vi "Destroy RawDataQs.vi"(8 "error in (no error)":errorcluster, 11 "DAQ":refnum<class "DAQ.lvclass">) -> (0 "error out":errorcluster, 3 "DAQ":refnum<class "DAQ.lvclass">)   [LabVIEW 2022 SP3, in "DAQ.lvclass"]
doc: "Developed by Kevin Thompson\nkevin@thompsonengineering.net\n\nCopyright 2018-2020\nThompson Engineering, LLC"
uses:
  DAQ.lvclass
  DAQ.lvclass/DAQ.ctl
  Process/ProcessSupport/TD local raw AI Data--cluster.ctl
  Support/DataQueues/DataTypes/DataQ SelectType--enum.ctl
  Support/DataQueues/DataQueues.lvclass
  DataTypes/Dependency--cluster.ctl
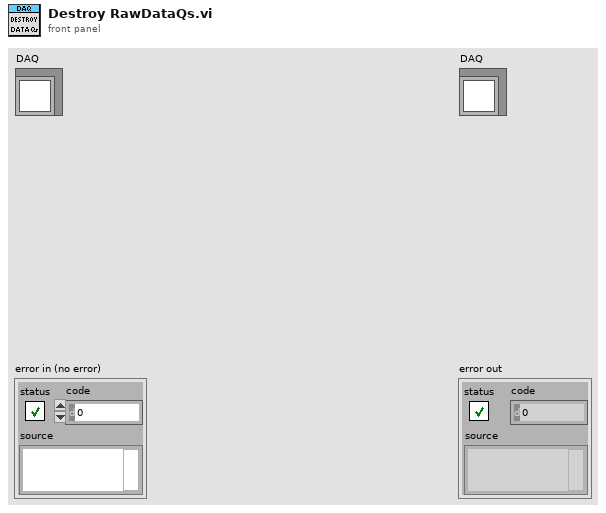
[diagram p1: front panel]
types:
  T1 = typedef "DAQ.lvclass/Dependency--cluster.ctl" = cluster{"DataQueues":refnum<class "DataQueues.lvclass">}
  T2 = typedef "DataQueues.lvclass/DataQ SelectType--enum.ctl" = enum16{"MainProcess", "LogEngine", "LocalDAQThread"}
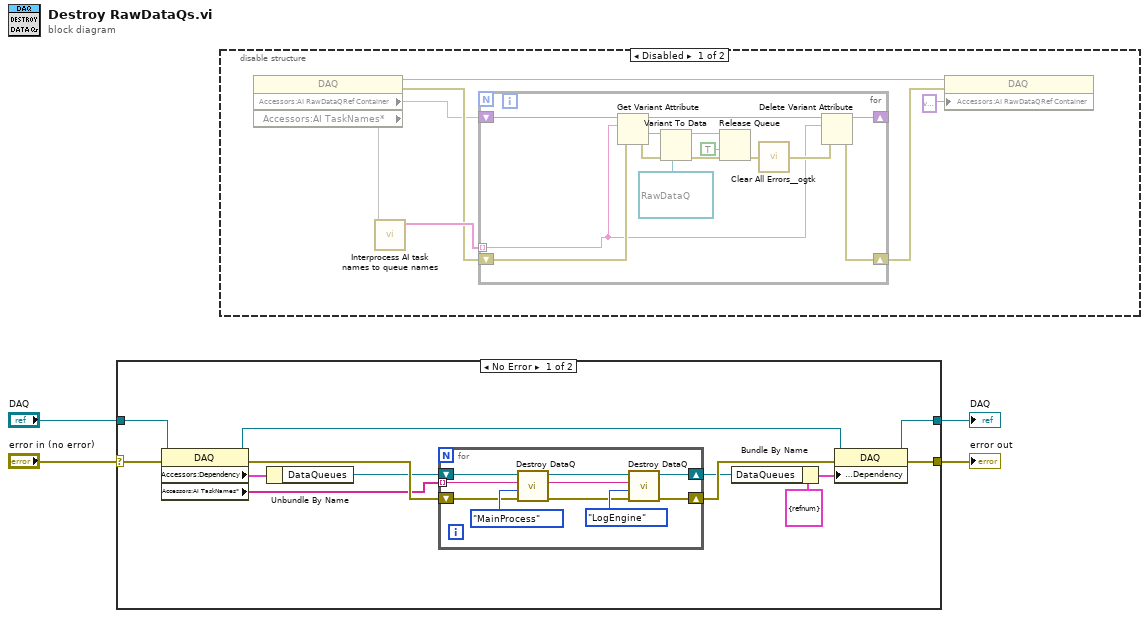
[diagram p0: block diagram]
diagram:
  n1 = case shown="No Error" "error in (no error)" {
    selector: "error in (no error)" -> [w17 w29]
    tunnel: [w16 w29] -> w3
    tunnel: [w11 w28] -> w1
    tunnel: "DAQ" -> [w10 w28]
    frame No Error {
      n2 = property class="DAQ"(reference=w10, error in=w17) -> (reference out=w12:refnum<class "DAQ.lvclass">, error out=w15:errorcluster, "Accessors:Dependency"=w9:T1, "Accessors:AI TaskNames*"=w13:string[])
      n3 = Unbundle By Name(w9) -> ("DataQueues"=w8:refnum<class "DataQueues.lvclass">)
      n4 = for {
        shift-right: [w23] -> w6
        shift-left: w8 -> [w27]
        shift-right: [w24] -> w14
        shift-left: w15 -> [w22]
        tunnel: w13 -> [w19] mode=indexing
        n5 = call "Destroy DataQ.vi"("error in (no error)"=w22, "Select"=DataQ_SelectType--enum."MainProcess", "TaskName"=w19, "DataQueues in"=w27) -> ("error out"=w20:errorcluster, "TaskName out"=w18:string, "DataQueues out"=w21:refnum<class "DataQueues.lvclass">)  [unwired: 5 in]
        n6 = call "Destroy DataQ.vi"("error in (no error)"=w20, "Select"=DataQ_SelectType--enum."LogEngine", "TaskName"=w18, "DataQueues in"=w21) -> ("error out"=w24:errorcluster, "DataQueues out"=w23:refnum<class "DataQueues.lvclass">)  [unwired: 5 in, 1 out]
      }
      n7 = Bundle By Name(cluster=T1 {"DataQueues"=refnum} ("Dependency"), "DataQueues"=w6) -> (w5:T1)
      n8 = property class="DAQ"(reference=w12, error in=w14, "Accessors:Dependency"=w5) -> (reference out=w11:refnum<class "DAQ.lvclass">, error out=w16:errorcluster)
    }
    frame Error {
    }
  }
  "error out" <- w3
  "DAQ" <- w1
  n9 = disable-structure shown="Disabled" {
    frame Disabled {
      n10 = property class="DAQ"() -> (reference out=w32:refnum<class "DAQ.lvclass">, error out=w31:errorcluster, "Accessors:AI RawDataQRef Container"=w30, "Accessors:AI TaskNames*"=w35)  [unwired: 2 in]
      n11 = call "Interprocess AI task names to queue names.vi"("Accessors:AI TaskNames*"=w35) -> ("All Queues"=w36:string[])  [unwired: 8 in, 2 out]
      n12 = for {
        shift-right: [w49] -> w33
        shift-left: w31 -> [w39]
        shift-right: [w50] -> _
        shift-left: w30 -> [w48]
        tunnel: w36 -> [w37] mode=indexing
        n13 = Get Variant Attribute(Variant=w48, name=w37, error in=w39) -> (duplicate Variant=w47:variant, value=w45:variant, error out=w46:errorcluster)  [unwired: 1 in, 1 out]
        n14 = Variant To Data(error in=w46, type=refnum<queue> refnum ("queue out"), Variant=w45) -> (data=w43:refnum<queue>, error out=w44:errorcluster)
        n15 = Release Queue(queue=w43, force destroy? (F)=TRUE, error in (no error)=w44) -> (error out=w40:errorcluster)  [unwired: 2 out]
        n16 = call <userlib>:"Clear All Errors__ogtk.vi"("Error In"=w40) -> ("Error Out"=w38:errorcluster)  [unwired: 3 in]
        n17 = Delete Variant Attribute(4:w38, 6:w37, 7:w47) -> (0:w49:errorcluster, 3:w50:variant)  [unwired: 1 out]
      }
      n18 = property class="DAQ"(reference=w32, error in=w33, "Accessors:AI RawDataQRef Container"=variant) -> ()  [unwired: 2 out]
    }
    frame Enabled {
    }
  }
